vi "Lin Ver Daten zusammensammeln.vi"(1 "KommLoopTimer":u32, 5 "Aktionen Daten abholen":T2, 7 "Aktion Unterbrechen":T1, 11 "error in (no error)":errorcluster caption="Fehler (Eingang, kein Fehler)") -> (4 "Anzeige aktualisieren":bool, 6 "Aktionen Daten abholen":T2, 8 "Aktion Unterbrechen":T1, 10 "Zustand":string, 15 "error out":errorcluster caption="Fehler (Ausgang)")   [LabVIEW 2020, in "Linearisierung v2.lvlib" / "Linearity verification 1065-307.lvlib"]
uses:
  Linearity verification 1065-307.lvlib
  Daten abholen.ctl
  Gasteiler/Aktion unterbrechen.ctl
  Gasteiler/Aktion FGV Daten Abholung uebergebenctl.ctl
  Aktion FGV Stoerungen sammeln und auswerten.ctl
  Funktionstasten/Funktionstasten-Aktion.ctl
  Funktionstasten/Zustaende.ctl
  Seiten/FT-IR/Algebraic Modul/FGV Algebraic Aktionen.ctl
  Sprachverwaltung/FGV Aktion Tabelle zerlegen.ctl
  Seiten/FT-IR/FGV FT-IR Gasliste Aktionen.ctl
  Aktion Lin Daten aufarbeiten.ctl
  Gasteiler/AK-Komm Gasteiler/Aktionen AK Komm.ctl
  Gasteiler/Aktionen FGV Gasteiler Daten.ctl
  SpanEinstellungen/Aktion FGV GD Errors sammeln.ctl
  SpanEinstellungen/GD Info Cluster.ctl
  LIN ErrorCluster.ctl
  Gasteiler/AK-Komm Gasteiler/Alter Gasteiler/Aktionen AK Komm_ALT.ctl
  Gasteiler/Horiba/Aktion Befehl.ctl
  Gasteiler/Gasteiler Fehler.ctl
  Linearisierung v2.lvlib
  Funktionstasten/Funktionstasten.lvlib
  Allgemein/allgemeine Sub-VIs.lvlib
  Sprachverwaltung/Sprachverwaltung.lvlib
  Gasteiler/Gasteiler.lvlib
  Gasteiler/AK-Komm Gasteiler/AK Komm Gasteiler.lvlib
  Gasteiler/Horiba/Horiba GDC.lvlib
  Gasteiler/AK-Komm Gasteiler/Alter Gasteiler/Alter Gasteiler.lvlib
  Seiten/FT-IR/Algebraic Modul/Algebraic Modul.lvlib
  Seiten/FT-IR/FT-IR.lvlib
  SpanEinstellungen/SpanEinstellungen.lvlib
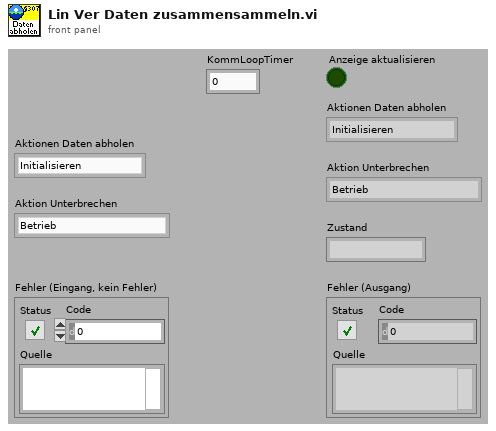
[diagram p1: front panel]
types:
  T1 = typedef "Linearisierung v2.lvlib/Gasteiler.lvlib/Aktion unterbrechen.ctl" = enum16{"Betrieb", "Unterbrechen", "Warten"}
  T2 = typedef "Linearisierung v2.lvlib/Daten abholen.ctl" = enum16{"Initialisieren", "Punkt aufschalten", "Warten", "Daten abholen", "Fertig", "Beenden", "Spülen", "Abbrechen"}
  T3 = typedef "Linearisierung v2.lvlib/Gasteiler.lvlib/Aktion FGV Daten Abholung uebergebenctl.ctl" = enum16{"lesen", "schreiben", "Anzeigebit löschen", "Status hinzufügen"}
  T4 = typedef "Linearisierung v2.lvlib/Aktion FGV Stoerungen sammeln und auswerten.ctl" = enum16{"init", "lesen", "error", "prüfen", "reset error", "abbrechen", "fortsetzen", "neustart", "Bedientasten reset"}
  T5 = typedef "Funktionstasten.lvlib/Zustaende.ctl" = enum16{"Standby", "Pause", "Eco", "Messen", "Kalibrieren", "Spülen Filter", "Spülen Leitung", "Umgebungsluft", "0-Gas", "Cal-Gas", "CG zu PNS", "-------------", "Init 1", "Init 2", "Init 3", "Init 4", "Messen vorbereiten", "Messen durchführen", "Exit"}
  T6 = typedef "Funktionstasten.lvlib/Funktionstasten-Aktion.ctl" = enum16{"Initialisieren", "Zustand setzen", "Taste gedrückt", "Fehler speichern", "Lesen", "Manuell", "Remote", "Bitparallel", "Samplepoint", "Zeit Prüfen", "reset Umschalten"}
  T7 = typedef "Linearisierung v2.lvlib/Gasteiler.lvlib/AK Komm Gasteiler.lvlib/Aktionen AK Komm.ctl" = enum16{"lesen", "initialisieren", "beenden", "Status", "SMAN", "SREM", "STBY", "ASTF", "ASTZ", "SLST", "AGAT", "EGAK", "AGAK", "AKAK", "ADRU", "SKOP", "SVSA", "SVSZ", "SONO", "SAIR", "SNOX", "ANOX", "SSPL", "SRUC", "SLIN", "ALST", "ETYP", "SVIO", "LCYL", "CCYL", "DCYL", "SCYL", "GCYL", "DRGV", "DRDC"}
  T8 = typedef "Linearisierung v2.lvlib/Aktion Lin Daten aufarbeiten.ctl" = enum16{"lesen", "Protkolldaten", "speichern", "laden", "EPA auswerten", "Tabelle schreiben", "Lin auswerten", "Tab init", "Stufentabelle", "EPA aktiviert", "Nachbehandlung laden", "Tabelle löschen", "Istwerte löschen", "Zeile löschen", "Zeile einfügen", "LIN aktiviert", "LIN/EPA aktiv laden", "EGAK Tab", "LIN übernehmen", "Tab init ohne Stufen"}
  T9 = typedef "FT-IR.lvlib/FGV FT-IR Gasliste Aktionen.ctl" = enum16{"lesen", "Gasliste FT-IR", "Gasliste ausgelesen", "laden", "speichern", "löschen"}
  T10 = typedef "Sprachverwaltung.lvlib/FGV Aktion Tabelle zerlegen.ctl" = enum16{"laden", "vereinzeln", "speichern"}
  T11 = typedef "FT-IR.lvlib/Algebraic Modul.lvlib/FGV Algebraic Aktionen.ctl" = enum16{"lesen", "laden", "speichern", "berechnen", "schreiben"}
  T12 = typedef "Linearisierung v2.lvlib/SpanEinstellungen.lvlib/GD Info Cluster.ctl" = cluster{"Wobei":string, "Status":string, "Errors":T13, "Empfangsdaten":string[], "Zeitstempel":string}
  T13 = typedef "Linearisierung v2.lvlib/LIN ErrorCluster.ctl" = cluster{"Störung Kommunikation":bool, "Pressure carrier gas":bool, "Pressure diluted gas":bool, "Outlet Pressure":bool, "SNOX before SAIR":bool, "Störung Gasteiler":bool}
  T14 = typedef "Linearisierung v2.lvlib/SpanEinstellungen.lvlib/Aktion FGV GD Errors sammeln.ctl" = enum16{"lesen", "init", "GD Infos sammeln", "Kalibrierinfos sammeln", "Test Data", "GD Infos selektiv sammeln"}
  T15 = typedef "Linearisierung v2.lvlib/Gasteiler.lvlib/Aktionen FGV Gasteiler Daten.ctl" = enum16{"lesen", "Gasteiler Daten", "Seriellen Param.", "MB-Endwert", "laden", "speichern", "Anforderung", "TCP", "Aufzeichnung Start"}
  T16 = typedef "Linearisierung v2.lvlib/Gasteiler.lvlib/AK Komm Gasteiler.lvlib/Alter Gasteiler.lvlib/Aktionen AK Komm_ALT.ctl" = enum16{"lesen", "initialisieren", "beenden", "SRES", "STBY", "SREM", "SMAN", "SLIN", "SLCH", "SLST", "SSPL", "AGAT", "ALST", "ASTZ", "ASTF", "AGAK", "EGAK"}
  T17 = typedef "Linearisierung v2.lvlib/Gasteiler.lvlib/Gasteiler Fehler.ctl" = cluster{"Pressure carrier gas":bool, "Pressure diluted gas":bool, "Outlet Pressure":bool, "SNOX before SAIR":bool}
  T18 = typedef "Linearisierung v2.lvlib/Gasteiler.lvlib/Horiba GDC.lvlib/Aktion Befehl.ctl" = enum16{"lesen", "initialisieren", "Beenden", "Standby", "GD/CC", "Info", "Flow", "Alarm", "GD parameter", "GD point", "Durchfluss", "Spuelen1", "Spuelen1 On", "Spuelen1Off", "Spuelen2", "Ventil-Abfrage", "Reset"}
  T19 = typedef "String - Ausgabefeld.ctl" = string
  T20 = typedef "Linearisierung v2.lvlib/Lin-Polynom Daten.ctl" = cluster{"Messgerät":string, "Kalibrator (Gasteiler)":string, "Bearbeiter/in":string, "Komponente":string, "Zeitstempel":timestamp, "F_max gefordert (%)":sgl, "F_max in %":sgl, "F_max in ppm":sgl, "Vorschlag Ordnung":i32, "Polynom OK":bool, "Polynomkoeff.":dbl[], "Prüfgas Konzentration":dbl, "Pfad EPA":string, "Pfad_LIN":string, "Gasnummer:":u8, "Komponentenauswahl":T21, "Verdünnungsgas":T23, "Zeitdauer Stufe":T24, "Anzahl Stufen":T24, "F_max in % EPA":sgl, "F_max in ppm EPA":sgl, "F_max in % LIN":sgl, "F_max in ppm LIN":sgl, "Punkte umkehren":bool, "EPA Optionsfeld":T25, "Autolin Hovacal":T26, "Spanfactors":sgl[], "Kalibrierauswahl":T27, "Conditions:":T28, "Gasflaschen Nr.:":string, "Bottle Accuracy":dbl, "Konfig Gasflasche":T29, "Gasflasche":T30, "HovaCAL Flow AutoLin":T31, "MFC Output":T32, "Gas Ablaufdatum":timestamp, "Lin Modus":T33, "zusätzliche Zeitdauer Erster Punkt":sgl, "Offsets":sgl[]}
  T21 = typedef "Linearisierung v2.lvlib/KomponentenArray.ctl" = cluster{"Komponente:":T22, "Konzentration":dbl}[]
  T22 = typedef "Auswahlfeld.ctl" = u16
  T23 = typedef "Linearisierung v2.lvlib/Gasteiler.lvlib/Prüfgas in.ctl" = u16
  T24 = typedef "Zahlen-Eingabefeld.ctl" = sgl
  T25 = typedef "Linearisierung v2.lvlib/EPA Optionsfeld.ctl" = enum32{"Istwert", "Rohwert", "Linearisierter Wert"}
  T26 = typedef "Linearisierung v2.lvlib/Gasteiler.lvlib/HovaCal.lvlib/AutoLin Hovacal.ctl" = enum32{"Keine Auswahl", "Optionsauswahl 1", "Optionsauswahl 2"}
  T27 = typedef "Linearisierung v2.lvlib/Kalibrieroption.ctl" = u16
  T28 = typedef "Linearisierung v2.lvlib/Linearity verification 1065-307.lvlib/Condition.ctl" = u16
  T29 = typedef "System Einstellungen V2.lvlib/Konfig Gasflasche.ctl" = bool
  T30 = typedef "System Einstellungen V2.lvlib/Gasflasche Auswahl.ctl" = u16
  T31 = typedef "Linearisierung v2.lvlib/Gasteiler.lvlib/HovaCAL_Interface.lvlib/Controls.lvlib/Flow Einstellung.ctl" = cluster{"HovaCAL Flow Input Cluster":dbl}
  T32 = typedef "Linearisierung v2.lvlib/Gasteiler.lvlib/HovaCAL_Interface.lvlib/Controls.lvlib/Pump state.ctl" = cluster{"Run":bool}
  T33 = typedef "CalGas Aufschaltung.lvlib/Lin Modus.ctl" = u16
  T34 = typedef "Linearisierung v2.lvlib/Gasteiler.lvlib/Stufen Tabelle.ctl" = string[][]
  T35 = typedef "Linearisierung v2.lvlib/GasteilerType.ctl" = u16
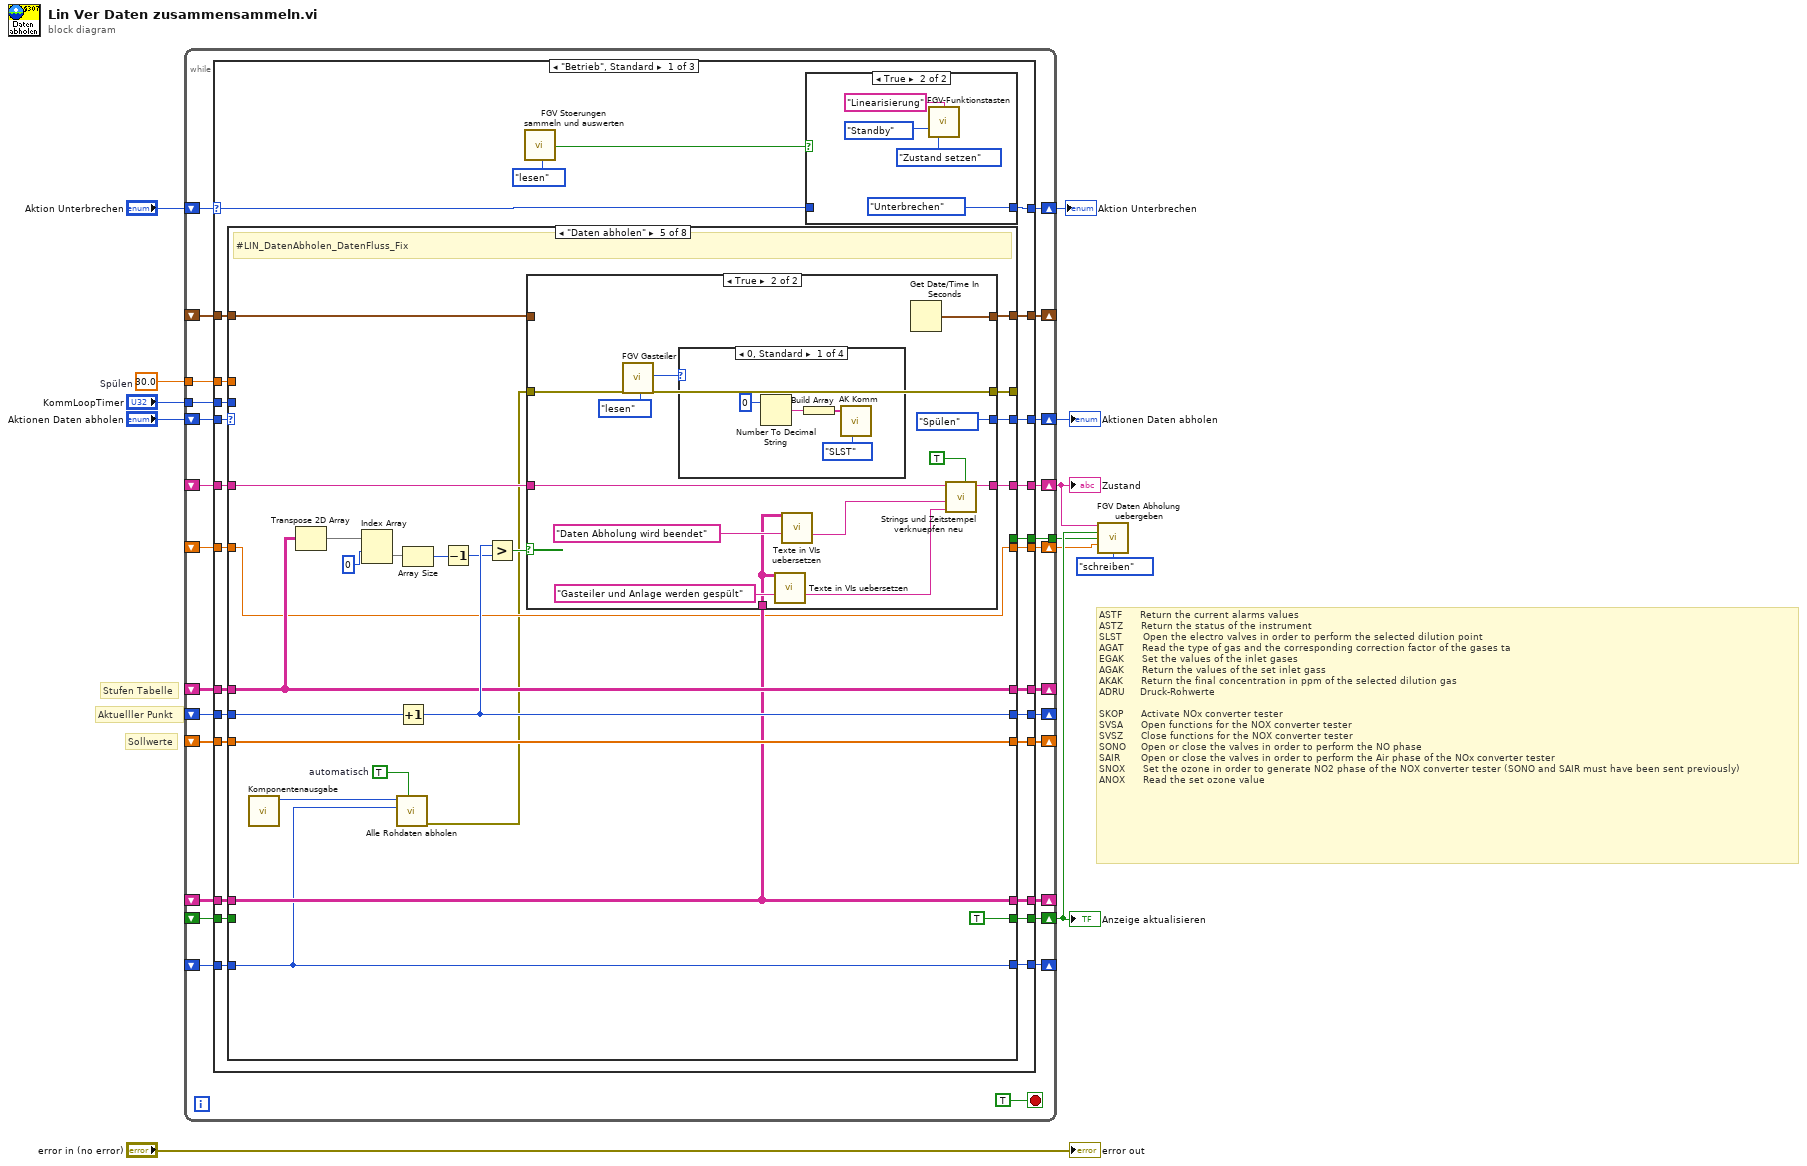
[diagram p0: block diagram]
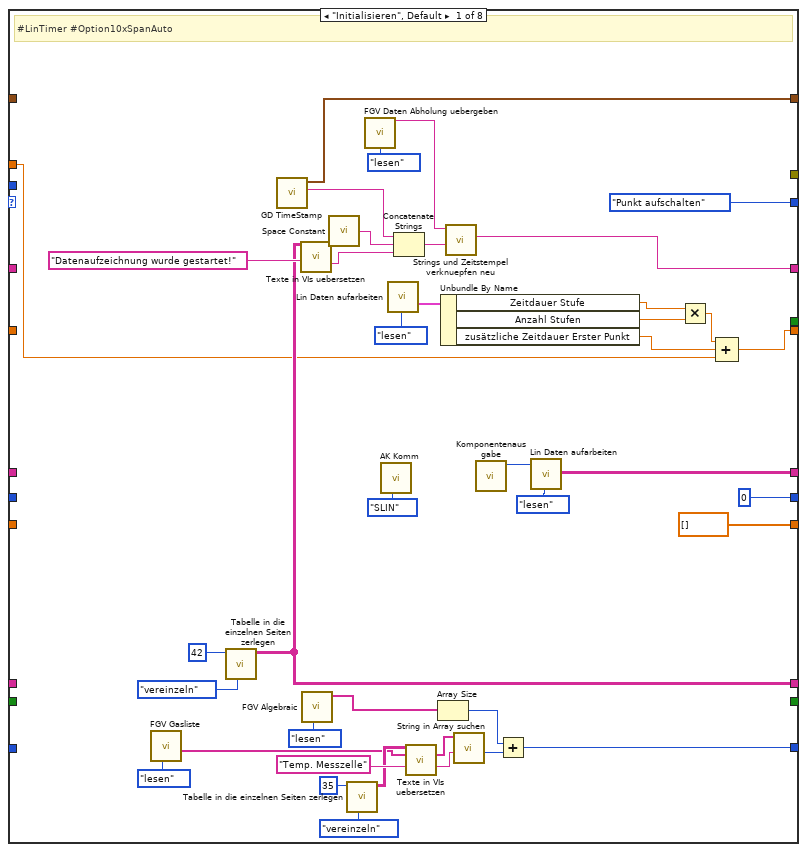
[diagram p3: hidden frame]
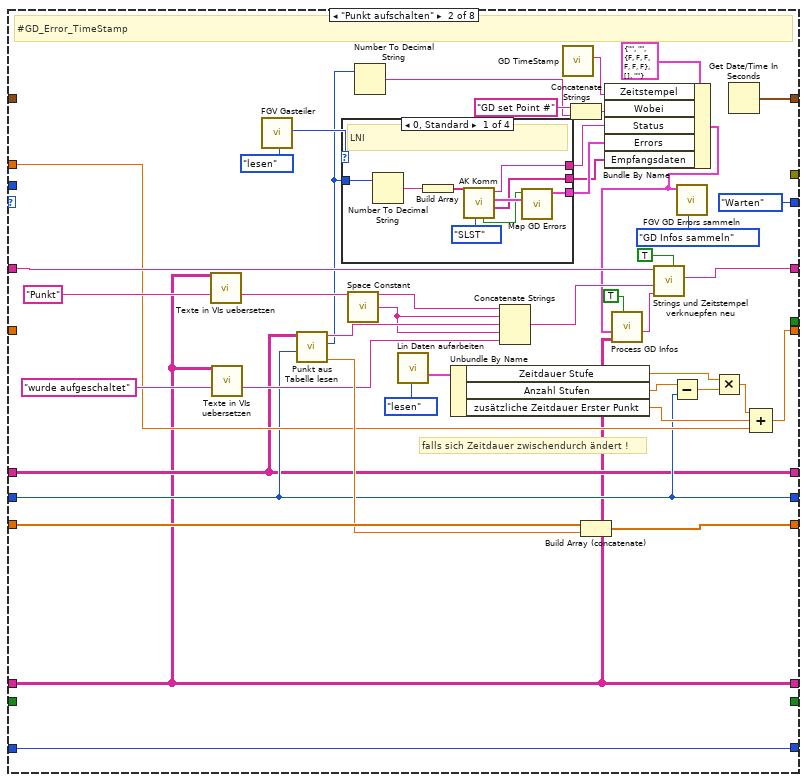
[diagram p4: hidden frame]
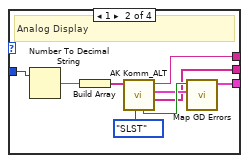
[diagram p5: hidden frame]
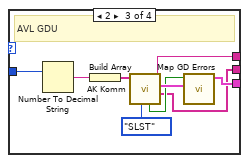
[diagram p6: hidden frame]
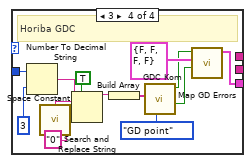
[diagram p7: hidden frame]
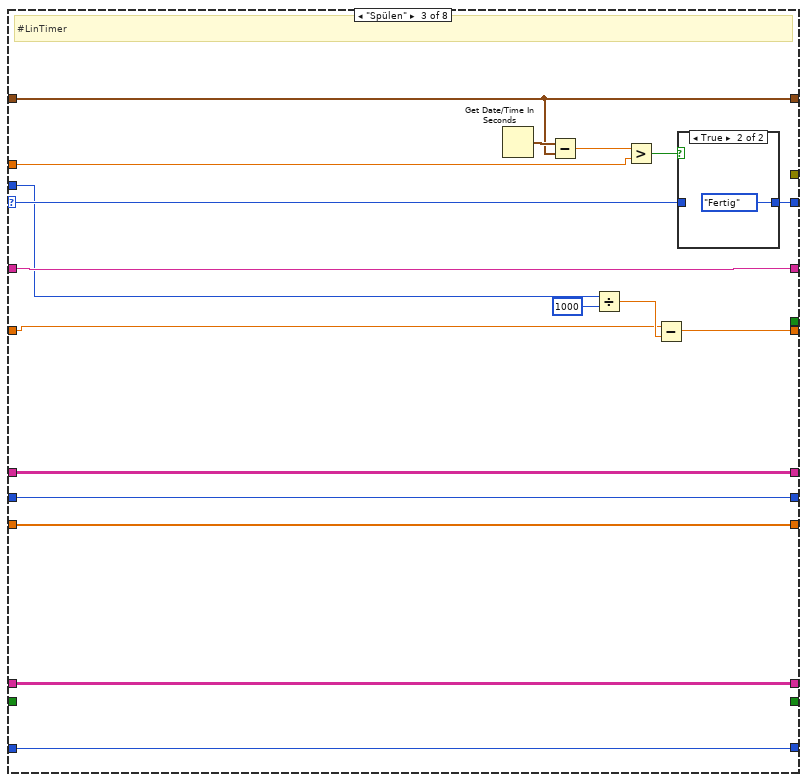
[diagram p8: hidden frame]
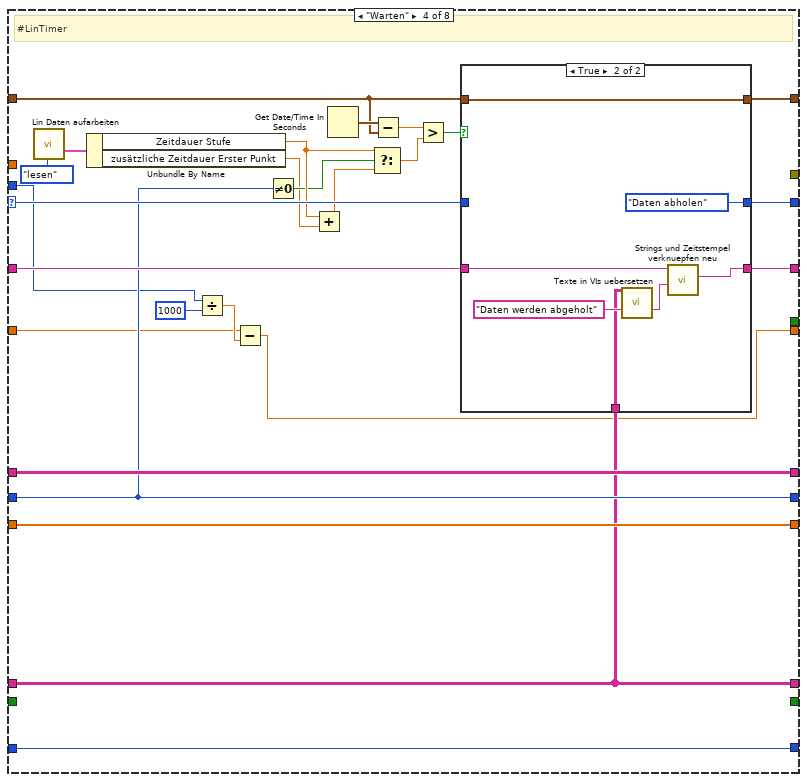
[diagram p10: hidden frame]
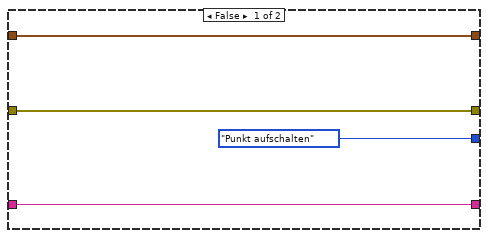
[diagram p12: hidden frame]
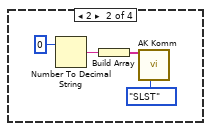
[diagram p13: hidden frame]
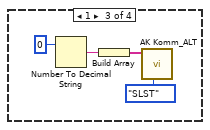
[diagram p14: hidden frame]
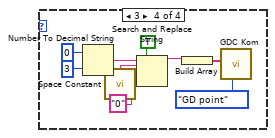
[diagram p15: hidden frame]
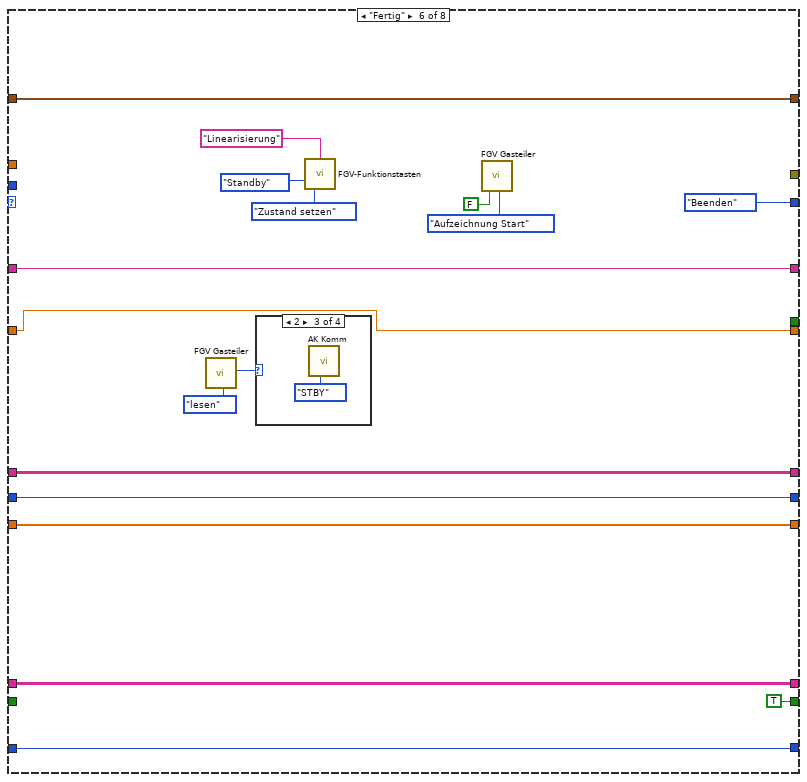
[diagram p16: hidden frame]
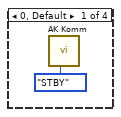
[diagram p17: hidden frame]
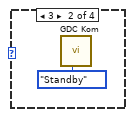
[diagram p18: hidden frame]
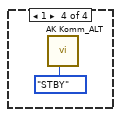
[diagram p19: hidden frame]
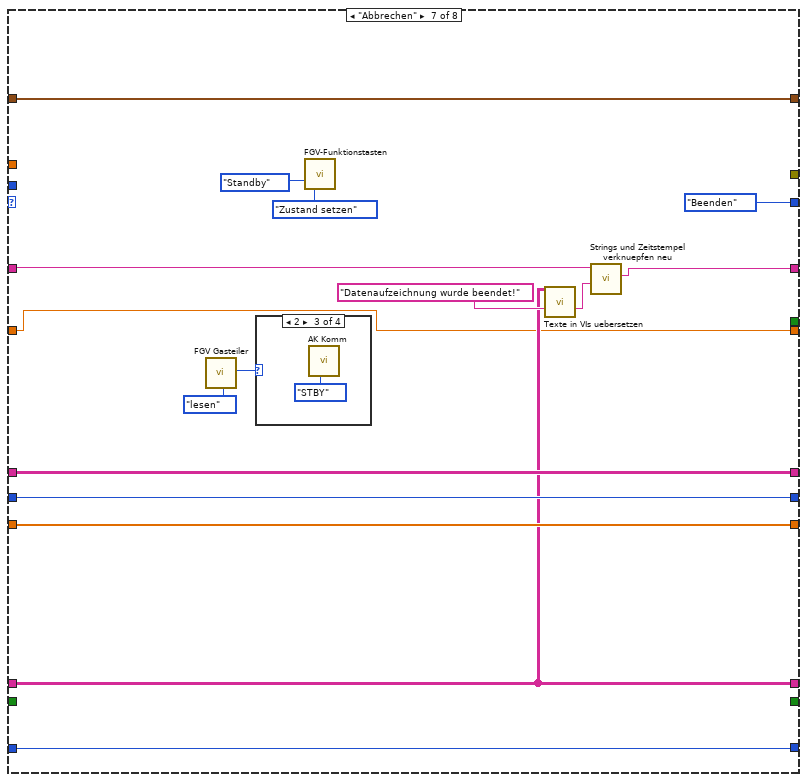
[diagram p20: hidden frame]
diagram:
  w2 = 30.0  # Spülen
  # "ASTF      Return the current alarms values\nASTZ      Return the status of the instrument \nSLST       Open the electro valves in order to perform the selected dilution point \nAGAT      Read the type of gas and the corresponding correction factor of the gases ta \nEGAK      Set the values of the inlet gases \nAGAK      Return the values of the set inlet gass \nAKAK      Return the final concentration in ppm of the selected dilution gas \nADRU     Druck-Rohwerte \n\nSKOP      Activate NOx converter tester \nSVSA      Open functions for the NOX converter tester \nSVSZ      Close functions for the NOX converter tester\nSONO     Open or close the valves in order to perform the NO phase\nSAIR       Open or close the valves in order to perform the Air phase of the NOx converter tester\nSNOX      Set the ozone in order to generate NO2 phase of the NOX converter tester (SONO and SAIR must have been sent previously)\nANOX      Read the set ozone value"
  # "Sollwerte"
  # "Stufen Tabelle"
  # "Aktuelller Punkt"
  n1 = while {
    shift-right: [w36] -> _
    shift-left: _ -> [w37]
    shift-right: [w32] -> w10
    shift-left: _ -> [w31]
    shift-right: [w29] -> _
    shift-left: _ -> [w34]
    shift-right: [w30] -> _
    shift-left: _ -> [w33]
    shift-right: [w27] -> _
    shift-left: _ -> [w26]
    shift-right: [w24] -> _
    shift-left: _ -> [w25]
    shift-right: [w23] -> w9
    shift-left: _ -> [w22]
    shift-right: [w21] -> _
    shift-left: _ -> [w20]
    shift-right: [w35] -> w12
    shift-left: "Aktionen Daten abholen" -> [w38]
    tunnel: [w19] -> w8
    shift-right: [w17] -> w6
    shift-left: "Aktion Unterbrechen" -> [w18]
    tunnel: w2 -> [w15]
    tunnel: "KommLoopTimer" -> [w13]
    shift-right: [w16] -> w4
    shift-left: _ -> [w14]
    stop <- TRUE stop-if-true
    n2 = case shown="\"Betrieb\", Standard" w18 {
      selector: w18 -> [w44 _ w387]
      tunnel: w38 -> [w65 w369 w389]
      tunnel: w37 -> [w64 w379 w400]
      tunnel: [w63 w379 w400] -> w36
      tunnel: [w62 w369 w399] -> w35
      tunnel: w34 -> [w61 w377 w397]
      tunnel: w33 -> [w60 w376 w396]
      tunnel: [w59 w370 w385] -> w32
      tunnel: w31 -> [w58 w371 w386]
      tunnel: [w57 w376 w396] -> w30
      tunnel: [w56 w377 w397] -> w29
      tunnel: [w55 w378 w398] -> w27
      tunnel: w26 -> [w54 w378 w398]
      tunnel: w25 -> [w53 w367 w384]
      tunnel: [w52 w367 w384] -> w24
      tunnel: [w51 w375 w395] -> w23
      tunnel: w22 -> [w50 w375 w395]
      tunnel: [w49 w374 w394] -> w21
      tunnel: w20 -> [w48 w374 w394]
      tunnel: [w47 _ _] -> w19
      tunnel: [w46 Aktion_unterbrechen."Warten" ("Aktion Unterbrechen") w388] -> w17
      tunnel: [w42 w364 w383] -> w16
      tunnel: w15 -> [w41 _ _]
      tunnel: w14 -> [w40 w364 w383]
      tunnel: w13 -> [w39 _ _]
      frame "Betrieb", Default {
        n3 = case shown="\"Daten abholen\"" w65 {
          selector: w65 -> [_ _ w202 w231 _ _ _ w359]
          tunnel: w64 -> [_ _ w204 w232 w260 w327 w347 w358]
          tunnel: [w72 w153 w204 w233 w259 w327 w347 w358] -> w63
          tunnel: [Daten_abholen."Punkt aufschalten" ("Aktionen Daten abholen") Daten_abholen."Warten" ("Aktionen Daten abholen") w209 w236 w272 Daten_abholen."Beenden" ("Aktionen Daten abholen") Daten_abholen."Beenden" ("Aktionen Daten abholen") w359] -> w62
          tunnel: w58 -> [_ w152 w208 w235 w265 w325 w337 w360]
          tunnel: [w74 w151 w208 w234 w264 w325 w336 w360] -> w59
          tunnel: w61 -> [_ w129 w210 w228 w271 w328 w348 w363]
          tunnel: w60 -> [_ w149 w207 w230 w258 w323 w344 w362]
          tunnel: [sgl[] [] ("Angehängtes Array") w147 w207 w230 w258 w323 w344 w362] -> w57
          tunnel: [0 ("Index") w129 w210 w228 w267 w328 w348 w363] -> w56
          tunnel: [w100 w121 w211 w229 w263 w324 w345 w361] -> w55
          tunnel: w54 -> [_ w121 w211 w229 w263 w324 w345 w361]
          tunnel: [w103 w115 w201 w223 w257 w319 w335 w357] -> w52
          tunnel: w53 -> [_ w115 w201 w223 w257 w319 w335 w357]
          tunnel: [_ _ _ _ TRUE TRUE _ TRUE] -> w51
          tunnel: w50 -> [_ _ _ _ _ _ _ _]
          tunnel: [w86 w137 w200 w220 w253 w317 w334 w356] -> w49
          tunnel: w48 -> [_ w137 w200 w220 w253 w317 w334 w356]
          tunnel: [_ _ _ _ _ _ _ TRUE] -> w47
          tunnel: [w78 w132 w196 w216 w254 w313 w333 w353] -> w42
          tunnel: w41 -> [w79 w131 w199 _ _ _ _ _]
          tunnel: w40 -> [_ _ w195 w217 w254 w313 w333 _]
          tunnel: w39 -> [_ _ w194 w215 _ _ _ _]
          tunnel: [_ _ _ _ w250 _ _ _] -> _
          frame "Initialisieren", Default {
            # "#LinTimer #Option10xSpanAuto"
            n4 = call "FGV Gasliste.vi"("Aktionen"=FGV_FT-IR_Gasliste_Aktionen."lesen") -> ("Aktuelle Gasliste gesamt"=w88:T19[])  [unwired: 8 in, 2 out]
            n5 = call "Tabelle in die einzelnen Seiten zerlegen.vi"("Aktion"=FGV_Aktion_Tabelle_zerlegen."vereinzeln", "Index (Seite)"=42) -> ("Sprachliste"=w103:string[][])  [unwired: 7 in, 2 out]
            n6 = call "GD TimeStamp.vi"() -> ("date/time string"=w71:string, "current time"=w72:timestamp)  [unwired: 10 in]
            n7 = call "Texte in VIs uebersetzen.vi"("Sprachliste"=w103, "String zum Übersetzen"="Datenaufzeichnung wurde gestartet!" ("String 1 hinzufügen")) -> ("String zum Übersetzen"=w104:string)  [unwired: 9 in, 4 out]
            n8 = call "FGV Algebraic.vi"("Aktionen Algebraic"=FGV_Algebraic_Aktionen."lesen") -> ("Namen"=w90:string[])  [unwired: 6 in, 4 out]
            n9 = call <vilib>:"Space Constant.vi"() -> ("String"=w109:string)
            n10 = call "Tabelle in die einzelnen Seiten zerlegen.vi"("Aktion"=FGV_Aktion_Tabelle_zerlegen."vereinzeln", "Index (Seite)"=35) -> ("Sprachliste"=w92:string[][])  [unwired: 7 in, 2 out]
            n11 = call "FGV Daten Abholung uebergeben.vi"("Aktion"=Aktion_FGV_Daten_Abholung_uebergebenctl."lesen") -> ("Zustand"=w76:string)  [unwired: 10 in, 4 out]
            n12 = call "AK Komm.vi"("Aktionen"=Aktionen_AK_Komm."SLIN") -> ()  [unwired: 4 in, 7 out]
            n13 = call "Lin Daten aufarbeiten.vi"("Aktionen"=Aktion_Lin_Daten_aufarbeiten."lesen") -> ("Lin-Polynom"=w84:T20)  [unwired: 16 in, 10 out]
            n14 = Concatenate Strings(w71, w109, w104) -> (w75:string)
            n15 = call "Texte in VIs uebersetzen.vi"("Sprachliste"=w92, "String-Array zum Übersetzen"=w88, "String zum Übersetzen"="Temp. Messzelle" ("Neues Element/Teil-Array")) -> ("String-Array zum Übersetzen"=w87:string[], "String zum Übersetzen"=w94:string)  [unwired: 8 in, 3 out]
            n16 = Array Size(array=w90) -> (size(s)=w96:i32)
            n17 = Unbundle By Name(w84) -> ("Zeitdauer Stufe"=w82:T24, "Anzahl Stufen"=w83:T24, "zusätzliche Zeitdauer Erster Punkt"=w80:sgl)
            n18 = call "Strings und Zeitstempel verknuepfen neu.vi"("String 1 hinzufügen"=w75, "Eingangs String"=w76) -> ("Verknüpfter String"=w74:string)  [unwired: 9 in]
            n19 = call "String in Array suchen.vi"("Nach String/Zeichen suchen (-)"=w94, "String-Array"=w87) -> ("Index"=w98:i32)  [unwired: 7 in, 2 out]
            n20 = call "Komponentenausgabe.vi"() -> ("Gaskomponente"=w99:T22)  [unwired: 8 in, 3 out]
            n21 = Add(x=w96, y=w98) -> (x+y=w86:i32)
            n22 = call "Lin Daten aufarbeiten.vi"("Index (Seite)"=w99, "Aktionen"=Aktion_Lin_Daten_aufarbeiten."lesen") -> ("Stufen Tabelle"=w100:T34)  [unwired: 15 in, 10 out]
            n23 = Multiply(x=w82, y=w83) -> (x*y=w81:T24)
            n24 = Compound Arithmetic op=unknown(w81, w80, w79) -> (w78:dbl)
          }
          frame "Punkt aufschalten" {
            # "falls sich Zeitdauer zwischendurch ändert !"
            # "#GD_Error_TimeStamp"
            n25 = call "Texte in VIs uebersetzen.vi"("Sprachliste"=w115, "String zum Übersetzen"="Punkt" ("String 1 hinzufügen")) -> ("String zum Übersetzen"=w142:string)  [unwired: 9 in, 4 out]
            n26 = call "Texte in VIs uebersetzen.vi"("Sprachliste"=w115, "String zum Übersetzen"="wurde aufgeschaltet" ("String")) -> ("String zum Übersetzen"=w139:string)  [unwired: 9 in, 4 out]
            n27 = call "FGV Gasteiler.vi"("Aktionen"=Aktionen_FGV_Gasteiler_Daten."lesen") -> ("Gasteiler Type"=w144:T35)  [unwired: 11 in, 7 out]
            n28 = call "Punkt aus Tabelle lesen.vi"("Index"=w129, "Stufen Tabelle"=w121) -> ("Sollwert"=w148:sgl, 2:"Punkt"=w118:i32, 3:"Punkt"=w150:string)  [unwired: 6 in, 1 out]
            n29 = case shown="0, Standard" w144 {
              tunnel: w118 -> [w161 w170 w179 w191]
              tunnel: [w157 w164 w174 w184] -> w125
              tunnel: [w156 w165 w173 _] -> w124
              tunnel: [w155 w163 w172 _] -> w123
              frame 0, Default {
                # "LNI"
                n30 = Number To Decimal String(number=w161) -> (decimal integer string=w162:string)  [unwired: 1 in]
                n31 = Build Array(w162) -> (w160:string[])
                n32 = call "AK Komm.vi"("Aktionen"=Aktionen_AK_Komm."SLST", "Daten"=w160) -> ("Empfangsdaten"=w155:string[], "Error"=w158:T17, "Status"=w156:string, "Störung Kommunikation"=w154:bool)  [unwired: 3 in, 3 out]
                n33 = call "Map GD Errors.vi"("Error"=w158, "Störung Kommunikation"=w154) -> ("LIN Errors-Cluster (Ausgang)"=w157:T13)  [unwired: 8 in, 1 out]
              }
              frame 1 {
                # "Analog Display"
                n34 = Number To Decimal String(number=w170) -> (decimal integer string=w171:string)  [unwired: 1 in]
                n35 = Build Array(w171) -> (w169:string[])
                n36 = call "AK Komm_ALT.vi"("Aktionen_ALT"=Aktionen_AK_Komm_ALT."SLST", "Daten"=w169) -> ("Empfangsdaten"=w163:string[], "Error"=w166:T17, "Status"=w165:string, "Störung Kommunikation"=w167:bool)  [unwired: 5 in, 1 out]
                n37 = call "Map GD Errors.vi"("Error"=w166, "Störung Kommunikation"=w167) -> ("LIN Errors-Cluster (Ausgang)"=w164:T13)  [unwired: 8 in, 1 out]
              }
              frame 2 {
                # "AVL GDU"
                n38 = Number To Decimal String(number=w179) -> (decimal integer string=w180:string)  [unwired: 1 in]
                n39 = Build Array(w180) -> (w178:string[])
                n40 = call "AK Komm.vi"("Aktionen"=Aktionen_AK_Komm."SLST", "Daten"=w178) -> ("Empfangsdaten"=w172:string[], "Error"=w176:T17, "Status"=w173:string, "Störung Kommunikation"=w175:bool)  [unwired: 3 in, 3 out]
                n41 = call "Map GD Errors.vi"("Error"=w176, "Störung Kommunikation"=w175) -> ("LIN Errors-Cluster (Ausgang)"=w174:T13)  [unwired: 8 in, 1 out]
              }
              frame 3 {
                # "Horiba GDC"
                n42 = Number To Decimal String(number=w191, width (-)=i16 3 ("Breite (-)")) -> (decimal integer string=w186:string)
                n43 = call <vilib>:"Space Constant.vi"() -> ("String"=w190:string)
                n44 = Search and Replace String(replace all?=TRUE ("Alle ersetzen? (F)"), input string=w186, search string=w190, replace string="0" ("Ersetzungs-String (\"\")")) -> (result string=w187:string)  [unwired: 4 in, 3 out]
                n45 = Build Array(w187) -> (w192:string[])
                n46 = call "GDC Kom.vi"("Befehl"=Aktion_Befehl."GD point", "Daten"=w192) -> ("Status (alarm)"=w181:bool, "Fehler"=w182:bool)  [unwired: 3 in, 5 out]
                n47 = call "Map GD Errors.vi"("Störung Gasteiler"=w181, "Error"=T17 {"Pressure carrier gas"=FALSE, "Pressure diluted gas"=FALSE, "Outlet Pressure"=FALSE, "SNOX before SAIR"=FALSE}, "Störung Kommunikation"=w182) -> ("LIN Errors-Cluster (Ausgang)"=w184:T13)  [unwired: 7 in, 1 out]
              }
            }
            n48 = call <vilib>:"Space Constant.vi"() -> ("String"=w140:string)
            n49 = Number To Decimal String(number=w118) -> (decimal integer string=w116:string)  [unwired: 1 in]
            n50 = call "Lin Daten aufarbeiten.vi"("Aktionen"=Aktion_Lin_Daten_aufarbeiten."lesen") -> ("Lin-Polynom"=w135:T20)  [unwired: 16 in, 10 out]
            n51 = Unbundle By Name(w135) -> ("Zeitdauer Stufe"=w114:T24, "Anzahl Stufen"=w113:T24, "zusätzliche Zeitdauer Erster Punkt"=w133:sgl)
            n52 = Concatenate Strings(w142, w140, w150, w140, w139) -> (w146:string)
            n53 = call "GD TimeStamp.vi"() -> ("date/time string"=w112:string)  [unwired: 10 in, 1 out]
            n54 = Concatenate Strings("GD set Point #" ("Status"), w116) -> (w117:string)
            n55 = Build Array (concatenate)(w149, w148) -> (w147:sgl[])
            n56 = Bundle By Name(cluster=T12 {"Wobei"="", "Status"="", "Errors"={"Störung Kommunikation"=FALSE, "Pressure carrier gas"=FALSE, "Pressure diluted gas"=FALSE, "Outlet Pressure"=FALSE, "SNOX before SAIR"=FALSE, "Störung Gasteiler"=FALSE}, "Empfangsdaten"=[], "Zeitstempel"=""} ("GD Info-Cluster in"), "Zeitstempel"=w112, "Wobei"=w117, "Status"=w124, "Errors"=w125, "Empfangsdaten"=w123) -> (w120:T12)
            n57 = call "Process GD Infos.vi"("show Status even if no Error"=TRUE, "Sprachliste"=w115, "GD Info-Cluster in"=w120) -> ("GD Infos"=w122:string)  [unwired: 6 in, 2 out]
            n58 = call "Strings und Zeitstempel verknuepfen neu.vi"("LF 1 -2"=TRUE, "String 2 hinzufügen"=w122, "String 1 hinzufügen"=w146, "Eingangs String"=w152) -> ("Verknüpfter String"=w151:string)  [unwired: 7 in]
            n59 = Subtract(x=w113, y=w129) -> (x-y=w130:T24)
            n60 = call "FGV GD Errors sammeln.vi"("Aktion"=Aktion_FGV_GD_Errors_sammeln."GD Infos sammeln", "GD Info-Cluster in"=w120) -> ()  [unwired: 7 in, 3 out]
            n61 = Multiply(x=w114, y=w130) -> (x*y=w134:T24)
            n62 = Get Date/Time In Seconds() -> (seconds since 1Jan1904=w153:timestamp)
            n63 = Compound Arithmetic op=unknown(w134, w133, w131) -> (w132:dbl)
          }
          frame "Spülen" {
            # "#LinTimer"
            n64 = Get Date/Time In Seconds() -> (seconds since 1Jan1904=w206:timestamp)
            n65 = Subtract(x=w206, y=w204) -> (x-y=w205:dbl)
            n66 = Divide(x=w194, y=u32 1000) -> (x/y=w197:dbl)
            n67 = Greater?(x=w205, y=w199) -> (0:w203:bool)
            n68 = Subtract(x=w195, y=w197) -> (x-y=w196:dbl)
            n69 = case shown="True" w203 {
              tunnel: [w212 Daten_abholen."Fertig" ("Aktionen Daten abholen")] -> w209
              tunnel: w202 -> [w212 _]
              frame False {
              }
              frame True {
              }
            }
          }
          frame "Warten" {
            # "#LinTimer"
            n70 = call "Lin Daten aufarbeiten.vi"("Aktionen"=Aktion_Lin_Daten_aufarbeiten."lesen") -> ("Lin-Polynom"=w221:T20)  [unwired: 16 in, 10 out]
            n71 = Unbundle By Name(w221) -> ("Zeitdauer Stufe"=w227:T24, "zusätzliche Zeitdauer Erster Punkt"=w214:sgl)
            n72 = Divide(x=w215, y=u32 1000) -> (x/y=w218:dbl)
            n73 = Subtract(x=w217, y=w218) -> (x-y=w216:dbl)
            n74 = Not Equal To 0?(x=w228) -> (x != 0?=w225:bool)
            n75 = Add(x=w227, y=w214) -> (x+y=w226:T24)
            n76 = Get Date/Time In Seconds() -> (seconds since 1Jan1904=w239:timestamp)
            n77 = Select(t=w227, s=w225, f=w226) -> (s? t:f=w224:T24)
            n78 = Subtract(x=w239, y=w232) -> (x-y=w238:dbl)
            n79 = Greater?(x=w238, y=w224) -> (0:w237:bool)
            n80 = case shown="True" w237 {
              tunnel: [w242 Daten_abholen."Daten abholen" ("Aktionen Daten abholen")] -> w236
              tunnel: w235 -> [w241 w249]
              tunnel: [w241 w248] -> w234
              tunnel: [w240 w246] -> w233
              tunnel: w232 -> [w240 w246]
              tunnel: w231 -> [w242 _]
              tunnel: w223 -> [_ w243]
              frame False {
                # "WARTEN!!!!"
              }
              frame True {
                n81 = call "Texte in VIs uebersetzen.vi"("Sprachliste"=w243, "String zum Übersetzen"="Daten werden abgeholt" ("String 1 hinzufügen")) -> ("String zum Übersetzen"=w244:string)  [unwired: 9 in, 4 out]
                n82 = call "Strings und Zeitstempel verknuepfen neu.vi"("String 1 hinzufügen"=w244, "Eingangs String"=w249) -> ("Verknüpfter String"=w248:string)  [unwired: 9 in]
              }
            }
          }
          frame "Daten abholen" {
            w255 = TRUE  # automatisch
            # "#LIN_DatenAbholen_DatenFluss_Fix"
            n83 = call "Komponentenausgabe.vi"() -> ("Gaskomponente"=w252:T22)  [unwired: 8 in, 3 out]
            n84 = Transpose 2D Array(2D array=w263) -> (transposed array=w262:T34)
            n85 = Index Array(array=w262, index (row)=0 ("Index (Zeile)")) -> (element=w268:string[])  [unwired: 1 in]
            n86 = call "Alle Rohdaten abholen.vi"("automatisch"=w255, "Temp. Messzelle G-nr."=w253, "Gasindex"=w252) -> ("error out"=w251:errorcluster)  [unwired: 7 in, 1 out]
            n87 = Increment(x=w271) -> (x+1=w267:i32)
            n88 = Array Size(array=w268) -> (size(s)=w269:i32)
            n89 = Decrement(x=w269) -> (x-1=w261:i32)
            n90 = Greater?(x=w267, y=w261) -> (0:w266:bool)
            n91 = case shown="True" w266 {
              tunnel: [Daten_abholen."Punkt aufschalten" ("Aktionen Daten abholen") Daten_abholen."Spülen" ("Aktionen Daten abholen")] -> w272
              tunnel: w265 -> [w275 w289]
              tunnel: [w275 w288] -> w264
              tunnel: w260 -> [w274 _]
              tunnel: [w274 w286] -> w259
              tunnel: w257 -> [_ w281]
              tunnel: w251 -> [w273 w278]
              tunnel: [w273 w277] -> w250
              frame False {
              }
              frame True {
                n92 = call "FGV Gasteiler.vi"("error in (no error)"=w278, "Aktionen"=Aktionen_FGV_Gasteiler_Daten."lesen") -> ("Gasteiler Type"=w287:T35, "error out"=w277:errorcluster)  [unwired: 10 in, 6 out]
                n93 = case shown="0, Standard" w287 {
                  frame 0, Default {
                    n94 = Number To Decimal String(number=0 ("Wert")) -> (decimal integer string=w293:string)  [unwired: 1 in]
                    n95 = Build Array(w293) -> (w292:string[])
                    n96 = call "AK Komm.vi"("Aktionen"=Aktionen_AK_Komm."SLST", "Daten"=w292) -> ()  [unwired: 3 in, 7 out]
                  }
                  frame 2 {
                    n97 = Number To Decimal String(number=0 ("Wert")) -> (decimal integer string=w297:string)  [unwired: 1 in]
                    n98 = Build Array(w297) -> (w296:string[])
                    n99 = call "AK Komm.vi"("Aktionen"=Aktionen_AK_Komm."SLST", "Daten"=w296) -> ()  [unwired: 3 in, 7 out]
                  }
                  frame 1 {
                    n100 = Number To Decimal String(number=0 ("Wert")) -> (decimal integer string=w302:string)  [unwired: 1 in]
                    n101 = Build Array(w302) -> (w301:string[])
                    n102 = call "AK Komm_ALT.vi"("Aktionen_ALT"=Aktionen_AK_Komm_ALT."SLST", "Daten"=w301) -> ()  [unwired: 5 in, 5 out]
                  }
                  frame 3 {
                    n103 = Number To Decimal String(number=0 ("Wert"), width (-)=i16 3 ("Breite (-)")) -> (decimal integer string=w305:string)
                    n104 = call <vilib>:"Space Constant.vi"() -> ("String"=w309:string)
                    n105 = Search and Replace String(replace all?=TRUE ("Alle ersetzen? (F)"), input string=w305, search string=w309, replace string="0" ("Ersetzungs-String (\"\")")) -> (result string=w306:string)  [unwired: 4 in, 3 out]
                    n106 = Build Array(w306) -> (w304:string[])
                    n107 = call "GDC Kom.vi"("Befehl"=Aktion_Befehl."GD point", "Daten"=w304) -> ()  [unwired: 3 in, 7 out]
                  }
                }
                n108 = call "Texte in VIs uebersetzen.vi"("Sprachliste"=w281, "String zum Übersetzen"="Gasteiler und Anlage werden gespült" ("String 2 hinzufügen")) -> ("String zum Übersetzen"=w284:string)  [unwired: 9 in, 4 out]
                n109 = call "Texte in VIs uebersetzen.vi"("Sprachliste"=w281, "String zum Übersetzen"="Daten Abholung wird beendet" ("String 1 hinzufügen")) -> ("String zum Übersetzen"=w282:string)  [unwired: 9 in, 4 out]
                n110 = Get Date/Time In Seconds() -> (seconds since 1Jan1904=w286:timestamp)
                n111 = call "Strings und Zeitstempel verknuepfen neu.vi"("LF 1 -2"=TRUE, "String 2 hinzufügen"=w284, "String 1 hinzufügen"=w282, "Eingangs String"=w289) -> ("Verknüpfter String"=w288:string)  [unwired: 7 in]
              }
            }
          }
          frame "Fertig" {
            n112 = call "FGV Gasteiler.vi"("Aktionen"=Aktionen_FGV_Gasteiler_Daten."lesen") -> ("Gasteiler Type"=w321:T35)  [unwired: 11 in, 7 out]
            n113 = case shown="2" w321 {
              frame 0, Default {
                n114 = call "AK Komm.vi"("Aktionen"=Aktionen_AK_Komm."STBY") -> ()  [unwired: 4 in, 7 out]
              }
              frame 3 {
                n115 = call "GDC Kom.vi"("Befehl"=Aktion_Befehl."Standby") -> ()  [unwired: 4 in, 7 out]
              }
              frame 2 {
                n116 = call "AK Komm.vi"("Aktionen"=Aktionen_AK_Komm."STBY") -> ()  [unwired: 4 in, 7 out]
              }
              frame 1 {
                n117 = call "AK Komm_ALT.vi"("Aktionen_ALT"=Aktionen_AK_Komm_ALT."STBY") -> ()  [unwired: 6 in, 5 out]
              }
            }
            n118 = call "FGV-Funktionstasten.vi"("Herkunft"="Linearisierung", "Zustand"=Zustaende."Standby", "Aktion"=Funktionstasten-Aktion."Zustand setzen") -> ()  [unwired: 5 in, 8 out]
            n119 = call "FGV Gasteiler.vi"("Aufzeichnung Start"=FALSE, "Aktionen"=Aktionen_FGV_Gasteiler_Daten."Aufzeichnung Start") -> ()  [unwired: 10 in, 8 out]
          }
          frame "Abbrechen" {
            n120 = call "FGV Gasteiler.vi"("Aktionen"=Aktionen_FGV_Gasteiler_Daten."lesen") -> ("Gasteiler Type"=w342:T35)  [unwired: 11 in, 7 out]
            n121 = case shown="2" w342 {
              frame 0, Default {
                n122 = call "AK Komm.vi"("Aktionen"=Aktionen_AK_Komm."STBY") -> ()  [unwired: 4 in, 7 out]
              }
              frame 3 {
                n123 = call "GDC Kom.vi"("Befehl"=Aktion_Befehl."Standby") -> ()  [unwired: 4 in, 7 out]
              }
              frame 2 {
                n124 = call "AK Komm.vi"("Aktionen"=Aktionen_AK_Komm."STBY") -> ()  [unwired: 4 in, 7 out]
              }
              frame 1 {
                n125 = call "AK Komm_ALT.vi"("Aktionen_ALT"=Aktionen_AK_Komm_ALT."STBY") -> ()  [unwired: 6 in, 5 out]
              }
            }
            n126 = call "FGV-Funktionstasten.vi"("Zustand"=Zustaende."Standby", "Aktion"=Funktionstasten-Aktion."Zustand setzen") -> ()  [unwired: 6 in, 8 out]
            n127 = call "Texte in VIs uebersetzen.vi"("Sprachliste"=w335, "String zum Übersetzen"="Datenaufzeichnung wurde beendet!" ("String 1 hinzufügen")) -> ("String zum Übersetzen"=w338:string)  [unwired: 9 in, 4 out]
            n128 = call "Strings und Zeitstempel verknuepfen neu.vi"("String 1 hinzufügen"=w338, "Eingangs String"=w337) -> ("Verknüpfter String"=w336:string)  [unwired: 9 in]
          }
          frame "Beenden" {
            w353 = sgl 0.0  # Restlaufzeit
            # "#LinTimer"
          }
        }
        n129 = call "FGV Stoerungen sammeln und auswerten.vi"("Aktion"=Aktion_FGV_Stoerungen_sammeln_und_auswerten."lesen") -> ("Error"=w43:bool)  [unwired: 12 in, 6 out]
        n130 = case shown="True" w43 {
          tunnel: [w66 Aktion_unterbrechen."Unterbrechen" ("Aktion Unterbrechen")] -> w46
          tunnel: w44 -> [w66 _]
          frame False {
          }
          frame True {
            n131 = call "FGV-Funktionstasten.vi"("Herkunft"="Linearisierung", "Zustand"=Zustaende."Standby", "Aktion"=Funktionstasten-Aktion."Zustand setzen") -> ()  [unwired: 5 in, 8 out]
          }
        }
      }
      frame "Unterbrechen" {
        n132 = call "FGV Gasteiler.vi"("Aktionen"=Aktionen_FGV_Gasteiler_Daten."lesen") -> ("Gasteiler Type"=w365:T35)  [unwired: 11 in, 7 out]
        n133 = case shown="3" w365 {
          frame 0, Default {
            n134 = call "AK Komm.vi"("Aktionen"=Aktionen_AK_Komm."STBY") -> ()  [unwired: 4 in, 7 out]
          }
          frame 3 {
            n135 = call "GDC Kom.vi"("Befehl"=Aktion_Befehl."Standby") -> ()  [unwired: 4 in, 7 out]
          }
          frame 1 {
            n136 = call "AK Komm_ALT.vi"("Aktionen_ALT"=Aktionen_AK_Komm_ALT."STBY") -> ()  [unwired: 6 in, 5 out]
          }
        }
        n137 = call "Texte in VIs uebersetzen.vi"("Sprachliste"=w367, "String zum Übersetzen"="Datenaufzeichnung wurde aufgrund eines Fehlers angehalten." ("String 1 hinzufügen")) -> ("String zum Übersetzen"=w372:string)  [unwired: 9 in, 4 out]
        n138 = call "Strings und Zeitstempel verknuepfen neu.vi"("String 1 hinzufügen"=w372, "Eingangs String"=w371) -> ("Verknüpfter String"=w370:string)  [unwired: 9 in]
      }
      frame "Warten" {
        n139 = call "FGV Stoerungen sammeln und auswerten.vi"("Aktion"=Aktion_FGV_Stoerungen_sammeln_und_auswerten."lesen") -> ("Neustart"=w391:bool, "Abbrechen"=w392:bool, "Fortsetzen"=w390:bool)  [unwired: 12 in, 4 out]
        n140 = case shown="False" w392 {
          tunnel: [Daten_abholen."Abbrechen" ("Aktionen Daten abholen") w413] -> w399
          tunnel: w391 -> [_ w412]
          tunnel: w390 -> [_ w411]
          tunnel: w389 -> [_ w410]
          tunnel: [Aktion_unterbrechen."Betrieb" ("Aktion Unterbrechen") w409] -> w388
          tunnel: w387 -> [_ w408]
          tunnel: w386 -> [w401 w407]
          tunnel: [w401 w406] -> w385
          tunnel: w384 -> [_ w405]
          frame True {
            # "Abbrechen"
            n141 = call "FGV Stoerungen sammeln und auswerten.vi"("Aktion"=Aktion_FGV_Stoerungen_sammeln_und_auswerten."Bedientasten reset") -> ()  [unwired: 12 in, 7 out]
          }
          frame False {
            # "Abbrechen"
            n142 = case shown="True" w412 {
              tunnel: [Daten_abholen."Initialisieren" ("Aktionen Daten abholen") w444] -> w413
              tunnel: w411 -> [_ w443]
              tunnel: w410 -> [_ w440]
              tunnel: [Aktion_unterbrechen."Betrieb" ("Aktion Unterbrechen") w442] -> w409
              tunnel: w408 -> [_ w441]
              tunnel: w407 -> [w424 w439]
              tunnel: [w423 w438] -> w406
              tunnel: w405 -> [w422 w437]
              tunnel: [w414 _] -> _
              frame True {
                # "Neustart"
                n143 = call "Lin Daten aufarbeiten.vi"("Aktionen"=Aktion_Lin_Daten_aufarbeiten."lesen") -> ("Lin-Polynom"=w421:T20)  [unwired: 16 in, 10 out]
                n144 = Unbundle By Name(w421) -> ("Lin Modus"=w419:T33)
                n145 = case shown="1, Standard" w419 {
                  tunnel: [Zustaende."Cal-Gas" ("Zustand") Zustaende."Messen" ("Zustand") Zustaende."CG zu PNS" ("Zustand")] -> w418
                  frame 1, Default {
                    # "Cal Gas to Samplepoint"
                  }
                  frame 2 {
                    # "Measure"
                  }
                  frame 0 {
                    # "Cal Gas to PNS"
                  }
                }
                n146 = call "FGV-Funktionstasten.vi"("Herkunft"="Linearisierung", "Zustand"=w418, "Aktion"=Funktionstasten-Aktion."Zustand setzen") -> ("Fehler steht an"=w416:bool)  [unwired: 5 in, 7 out]
                n147 = disable-structure shown="Deaktiviert" {
                  disable-tunnel: [w432 _] -> w415
                  disable-tunnel: w416 -> [w431 _]
                  frame Disabled {
                    # "UNKLAR !"
                    n148 = call "warten.vi"("Datenfluss"=w431, "Zu wartende ms"=u32 3000) -> ("error out"=w432:errorcluster)  [unwired: 8 in, 1 out]
                  }
                  frame Enabled {
                  }
                }
                n149 = call "Texte in VIs uebersetzen.vi"("Sprachliste"=w422, "String zum Übersetzen"="Datenaufzeichnung wird neu gestartet." ("String 1 hinzufügen")) -> ("String zum Übersetzen"=w425:string)  [unwired: 9 in, 4 out]
                n150 = call "Strings und Zeitstempel verknuepfen neu.vi"("String 1 hinzufügen"=w425, "Eingangs String"=w424) -> ("Verknüpfter String"=w423:string)  [unwired: 9 in]
                n151 = call "FGV Stoerungen sammeln und auswerten.vi"("error in (no error)"=w415, "Aktion"=Aktion_FGV_Stoerungen_sammeln_und_auswerten."Bedientasten reset") -> ("error out"=w414:errorcluster)  [unwired: 11 in, 6 out]
              }
              frame False {
                # "Neustart"
                n152 = case shown="True" w443 {
                  tunnel: [w447 Daten_abholen."Punkt aufschalten" ("Aktionen Daten abholen")] -> w444
                  tunnel: w440 -> [w447 _]
                  tunnel: [w446 Aktion_unterbrechen."Betrieb" ("Aktion Unterbrechen")] -> w442
                  tunnel: w441 -> [w446 _]
                  tunnel: w439 -> [w445 w459]
                  tunnel: [w445 w458] -> w438
                  tunnel: w437 -> [_ w457]
                  tunnel: [_ w450] -> _
                  frame False {
                    # "Fortsetzen"
                  }
                  frame True {
                    # "Fortsetzen"
                    n153 = call "Lin Daten aufarbeiten.vi"("Aktionen"=Aktion_Lin_Daten_aufarbeiten."lesen") -> ("Lin-Polynom"=w456:T20)  [unwired: 16 in, 10 out]
                    n154 = Unbundle By Name(w456) -> ("Lin Modus"=w454:T33)
                    n155 = case shown="0" w454 {
                      tunnel: [Zustaende."Cal-Gas" ("Zustand") Zustaende."Cal-Gas" ("Zustand") Zustaende."Messen" ("Zustand") Zustaende."Cal-Gas" ("Zustand")] -> w453
                      frame 0 {
                        # "Cal Gas to PNS"
                      }
                      frame 1, Default {
                        # "Cal Gas to Samplepoint"
                      }
                      frame 2 {
                        # "Measure"
                      }
                      frame 3 {
                        # "Gasdivider"
                      }
                    }
                    n156 = call "FGV-Funktionstasten.vi"("Herkunft"="Linearisierung", "Zustand"=w453, "Aktion"=Funktionstasten-Aktion."Zustand setzen") -> ("Fehler steht an"=w451:bool)  [unwired: 5 in, 7 out]
                    n157 = disable-structure shown="Deaktiviert" {
                      disable-tunnel: [w467 _] -> w449
                      disable-tunnel: w451 -> [w466 _]
                      frame Disabled {
                        # "UNKLAR !"
                        n158 = call "warten.vi"("Datenfluss"=w466, "Zu wartende ms"=u32 3000) -> ("error out"=w467:errorcluster)  [unwired: 8 in, 1 out]
                      }
                      frame Enabled {
                      }
                    }
                    n159 = call "Texte in VIs uebersetzen.vi"("Sprachliste"=w457, "String zum Übersetzen"="Datenaufzeichnung wird fortgesetzt." ("String 1 hinzufügen")) -> ("String zum Übersetzen"=w460:string)  [unwired: 9 in, 4 out]
                    n160 = call "Strings und Zeitstempel verknuepfen neu.vi"("String 1 hinzufügen"=w460, "Eingangs String"=w459) -> ("Verknüpfter String"=w458:string)  [unwired: 9 in]
                    n161 = call "AVL SLIN.vi"("error in (no error)"=w449) -> ("error out"=w448:errorcluster)  [unwired: 10 in]
                    n162 = call "FGV Stoerungen sammeln und auswerten.vi"("error in (no error)"=w448, "Aktion"=Aktion_FGV_Stoerungen_sammeln_und_auswerten."Bedientasten reset") -> ("error out"=w450:errorcluster)  [unwired: 11 in, 6 out]
                  }
                }
              }
            }
          }
        }
      }
    }
  }
  "Zustand" <- w10
  "Aktionen Daten abholen" <- w12
  "Anzeige aktualisieren" <- w9
  "Aktion Unterbrechen" <- w6
  n163 = call "FGV Daten Abholung uebergeben.vi"("Zustand"=w10, "Anzeige aktualisieren"=w9, "Beendet"=w8, "Restlaufzeit"=w4, "Aktion"=Aktion_FGV_Daten_Abholung_uebergebenctl."schreiben") -> ()  [unwired: 6 in, 5 out]
  "error out" <- "error in (no error)"
